vi "Add Pattern Script Header.vi"(8 "error in (no error)":errorcluster, 9 "Pattern Script Frame in":string, 10 "Pattern Name":string, 11 "BML Pattern Creater":refnum<class "BML Pattern Creater.lvclass">) -> (0 "error out":errorcluster, 2 "Pattern Script All out":string, 3 "BML Pattern Creater":refnum<class "BML Pattern Creater.lvclass">)   [LabVIEW 2018, in "BML Pattern Creater.lvlib" / "BML Pattern Creater.lvclass"]
uses:
  BML Pattern Creater.lvclass
  Interfaces/Protocol Interface.lvlibp/Interfaces/Protocol Interface/Pin State.ctl
  Interfaces/Protocol Interface.lvlibp/Interfaces/Protocol Interface/Protocol Interface.lvclass
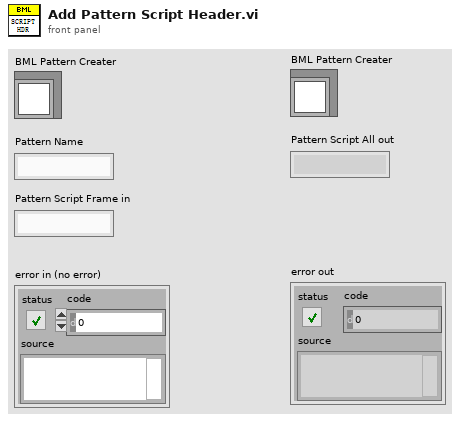
[diagram p1: front panel]
types:
  T1 = typedef "Protocol Interface.lvlibp/Protocol Interface.lvclass/Pin State.ctl" = enum16{"0", "1", "L", "H", "X", "V", "D", "M"}
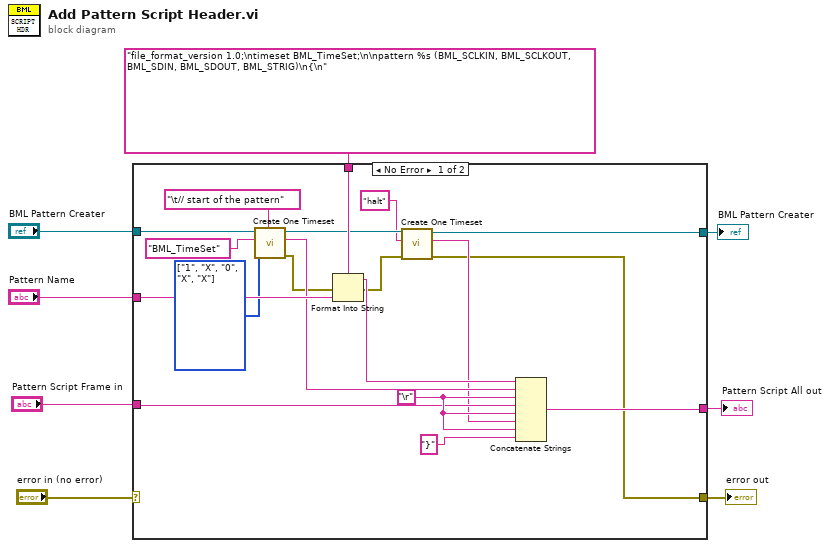
[diagram p0: block diagram]
diagram:
  n1 = case shown="No Error" "error in (no error)" {
    selector: "error in (no error)" -> [_ w29]
    tunnel: "Pattern Name" -> [w27 _]
    tunnel: "Pattern Script Frame in" -> [w17 _]
    tunnel: "file_format_version 1.0;\ntimeset BML_TimeSet;\n\npattern %s (BML_SCLKIN, BML_SCLKOUT, BML_SDIN, BML_SDOUT, BML_STRIG)\n{\n" -> [w23 _]
    tunnel: "BML Pattern Creater" -> [w22 w28]
    tunnel: [w12 w28] -> w3
    tunnel: [w10 _] -> w2
    tunnel: [w9 w29] -> w1
    frame No Error {
      w19 = T1[] [enum."1", enum."X", enum."0", enum."X", enum."X"] items=["0", "1", "L", "H", "X", "V", "D", "M"] ("Pin State")
      w26 = "\r"
      n2 = call-dynamic "Create One Timeset.vi"("Notes"="\t// start of the pattern", "Pin State"=w19, "opcode"="BML_TimeSet" ("timeset name"), "BML Pattern Creater in"=w22) -> ("error out"=w16:errorcluster, "string out"=w18:string, "BML Pattern Creater out"=w14:refnum<class "BML Pattern Creater.lvclass">)  [unwired: 5 in]
      n3 = Format Into String(format string=w23, error in=w16, w27) -> (resulting string=w24:string, error out=w15:errorcluster)  [unwired: 1 in]
      n4 = call-dynamic "Create One Timeset.vi"("error in (no error)"=w15, "opcode"="halt", "BML Pattern Creater in"=w14) -> ("error out"=w9:errorcluster, "string out"=w11:string, "BML Pattern Creater out"=w12:refnum<class "BML Pattern Creater.lvclass">)  [unwired: 6 in]
      n5 = Concatenate Strings(w24, w18, w26, w17, w26, w11, w26, "}") -> (w10:string)
    }
    frame Error {
    }
  }
  "error out" <- w1
  "Pattern Script All out" <- w2
  "BML Pattern Creater" <- w3
